vi "aggregator - viii - real - atomic.vi"(5 "aggregator action":T1, 7 "requested size":i32=20, 8 "number":dbl, 11 "state IN":T2={"Array "=[], "actual size"=0, "requested size"=20}) -> (0 "slope":dbl, 1 "interp average":dbl, 2 "mean":dbl, 3 "state OUT":T2={"Array "=[], "actual size"=0, "requested size"=20})   [LabVIEW 2021]
uses:
  interpolation state - real.ctl
  agregator -- action.ctl
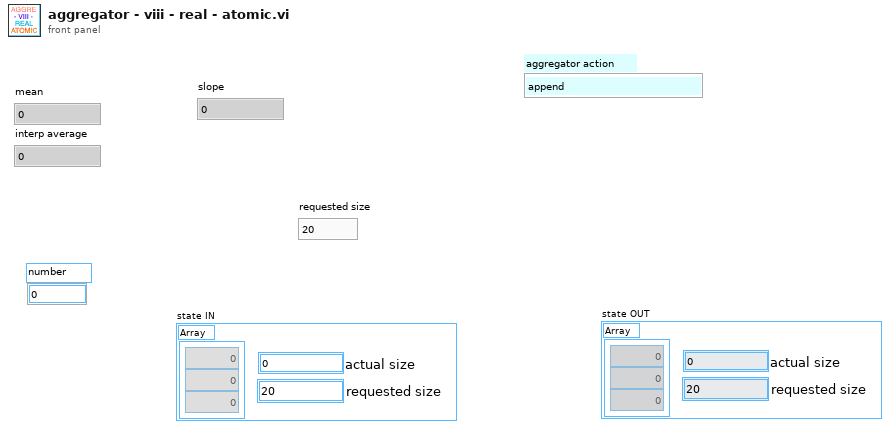
[diagram p1: front panel]
types:
  T1 = typedef "agregator -- action.ctl" = enum16{"append", "interpolate", "empty!", "force", "init", "scale", "read last"}
  T2 = typedef "interpolation state - real.ctl" = cluster{"Array ":dbl[], "actual size":i32, "requested size":i32}
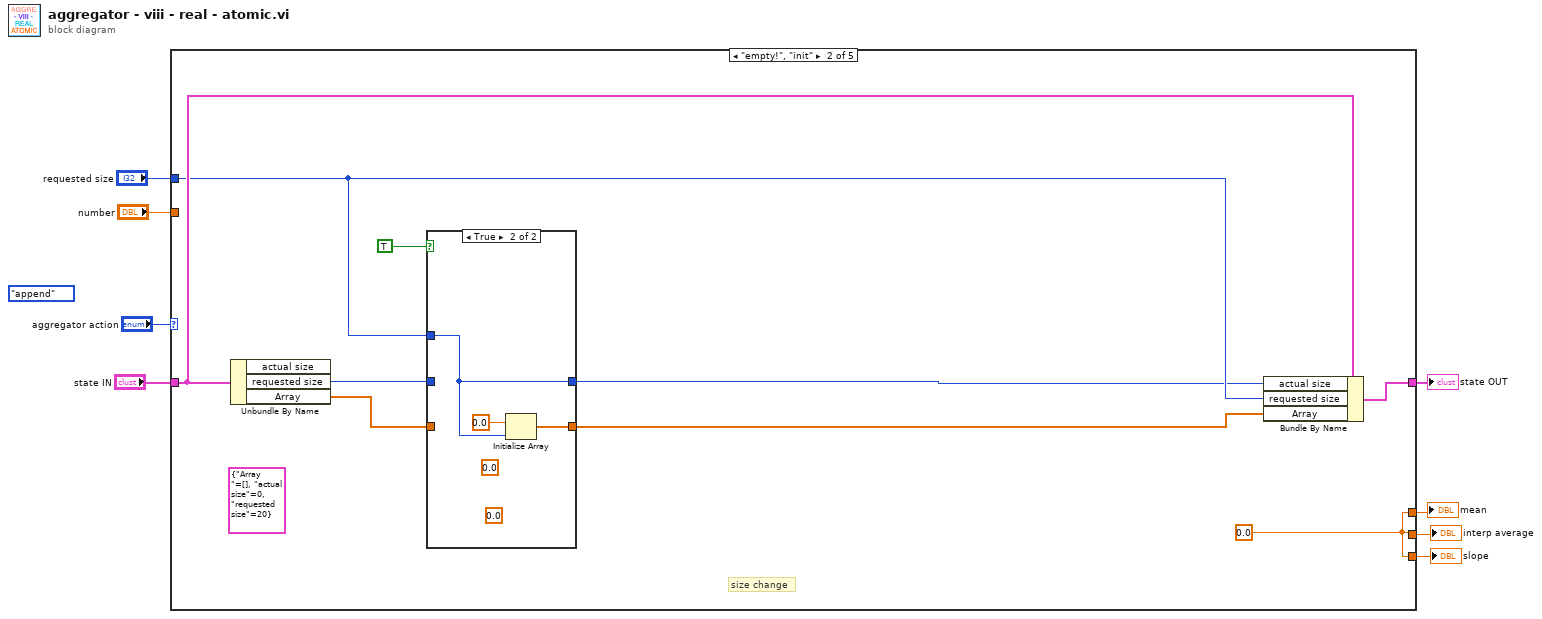
[diagram p0: block diagram]
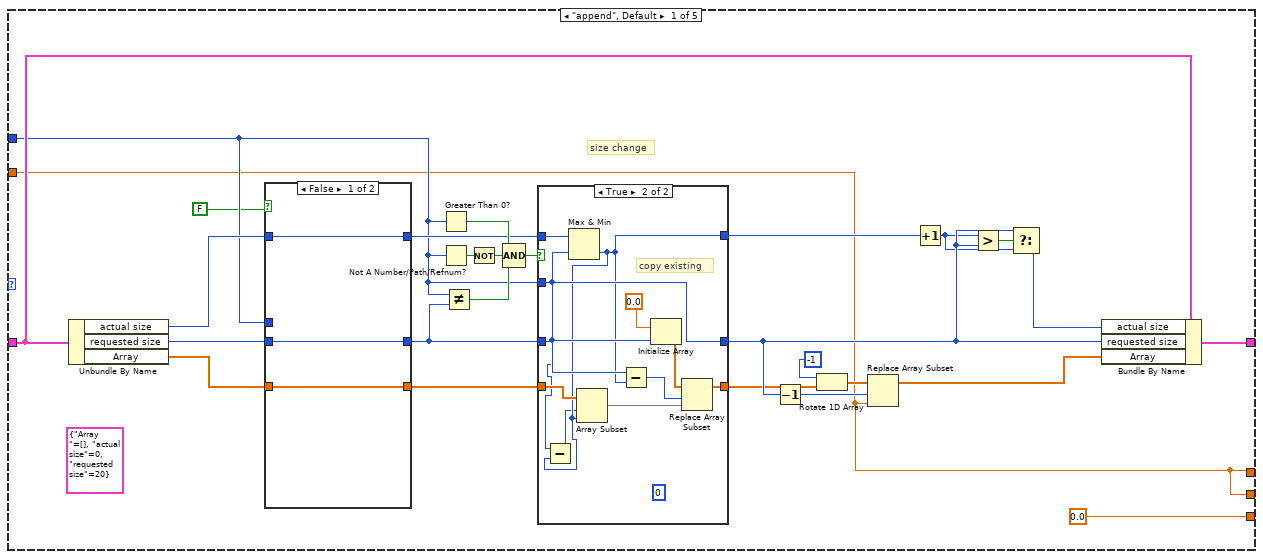
[diagram p2: hidden frame]
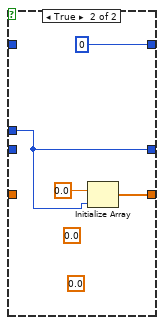
[diagram p4: hidden frame]
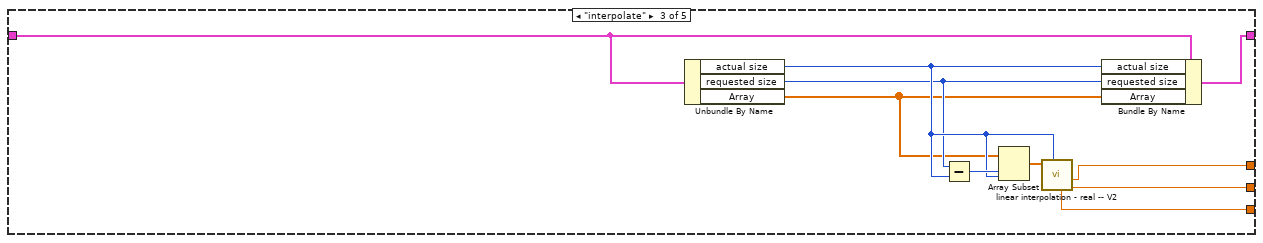
[diagram p6: hidden frame]
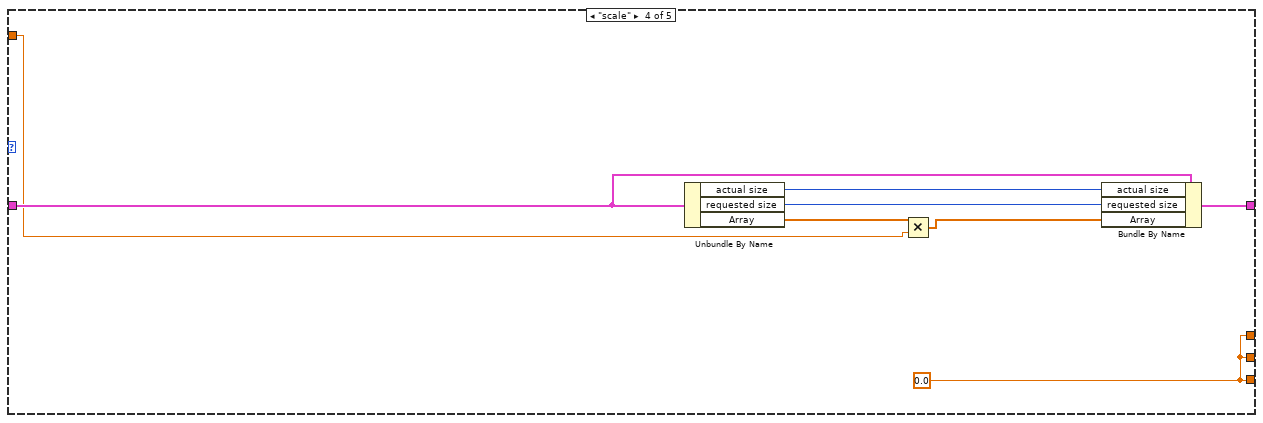
[diagram p7: hidden frame]
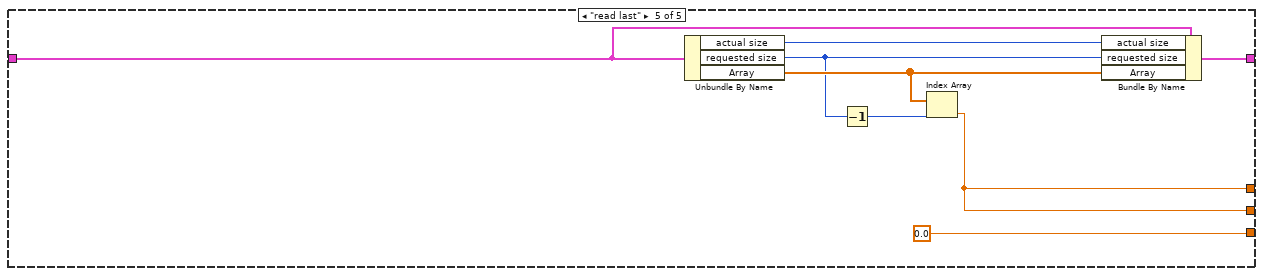
[diagram p8: hidden frame]
diagram:
  (unwired) agregator_--_action."append" ("aggregator action")
  n1 = case shown="\"empty!\", \"init\"" "aggregator action" {
    tunnel: [w9 w61 w80 w84 w89] -> w8
    tunnel: [w9 w61 w79 w84 w89] -> w7
    tunnel: [0.0 ("mean") w61 w78 w84 0.0 ("mean")] -> w6
    tunnel: [w32 w63 w77 w88 w96] -> w5
    tunnel: "state IN" -> [w31 w62 w76 w87 w95]
    tunnel: "number" -> [w9 _ _ w82 _]
    tunnel: "requested size" -> [w11 w58 _ _ _]
    frame "append", Default {
      (unwired) T2 {"Array "=[], "actual size"=0, "requested size"=20} ("Cluster")
      # "size change"
      n2 = Unbundle By Name(w31) -> ("actual size"=w34:i32, "requested size"=w35:i32, "Array"=w33:dbl[])
      n3 = case shown="False" FALSE {
        tunnel: w34 -> [w52 _]
        tunnel: [w52 0] -> w17
        tunnel: w33 -> [w50 _]
        tunnel: w11 -> [_ w53]
        tunnel: w35 -> [w51 _]
        tunnel: [w50 w54] -> w20
        tunnel: [w51 w53] -> w18
        frame False {
        }
        frame True {
          (unwired) 0.0
          (unwired) 0.0
          n4 = Initialize Array(0.0, w53) -> (w54:dbl[])
        }
      }
      n5 = Greater Than 0?(x=w11) -> (x > 0?=w24:bool)
      n6 = Not A Number/Path/Refnum?(number/path/refnum=w11) -> (NaN/Path/Refnum?=w25:bool)
      n7 = Not Equal?(x=w11, y=w18) -> (x != y?=w22:bool)
      n8 = Not(x=w25) -> (.not. x?=w23:bool)
      n9 = Compound Arithmetic op=AND(w24, w23, w22) -> (w21:bool)
      n10 = case shown="True" w21 {
        tunnel: [w38 w40] -> w16
        tunnel: w17 -> [w38 w48]
        tunnel: [w37 w44] -> w29
        tunnel: w18 -> [w37 w41]
        tunnel: [w36 w47] -> w19
        tunnel: w20 -> [w36 w43]
        tunnel: w11 -> [_ w44]
        frame False {
        }
        frame True {
          (unwired) 0 ("disabled index (col)")
          # "copy existing"
          n11 = Max & Min(x=w48, y=w44) -> (min(x,y)=w40:i32)  [unwired: 1 out]
          n12 = Subtract(x=w41, y=w40) -> (x-y=w39:i32)
          n13 = Array Subset(array=w43, index=w39, length=w40) -> (w42:dbl[])
          n14 = Subtract(x=w44, y=w40) -> (x-y=w45:i32)
          n15 = Initialize Array(0.0, w44) -> (w46:dbl[])
          n16 = Replace Array Subset(array=w46, new element=w42, index=w45) -> (w47:dbl[])
        }
      }
      n17 = Decrement(x=w29) -> (x-1=w14:i32)
      n18 = Rotate 1D Array(1:w19, 2:-1 ("n")) -> (0:w13:dbl[])
      n19 = Replace Array Subset(array=w13, new element=w9, index=w14) -> (w28:dbl[])
      n20 = Increment(x=w16) -> (x+1=w26:i32)
      n21 = Greater?(x=w26, y=w29) -> (0:w27:bool)
      n22 = Select(t=w29, s=w27, f=w26) -> (s? t:f=w30:i32)
      n23 = Bundle By Name(cluster=w31, "actual size"=w30, "requested size"=w29, "Array"=w28) -> (w32:T2)
    }
    frame "empty!", "init" {
      w61 = 0.0 ("mean")
      (unwired) T2 {"Array "=[], "actual size"=0, "requested size"=20} ("Cluster")
      # "size change"
      n24 = Unbundle By Name(w62) -> ("requested size"=w65:i32, "Array"=w64:dbl[])  [unwired: 1 out]
      n25 = case shown="True" TRUE {
        tunnel: w64 -> [w66 _]
        tunnel: w58 -> [_ w68]
        tunnel: w65 -> [w67 _]
        tunnel: [w66 w69] -> w59
        tunnel: [w67 w68] -> w57
        frame False {
        }
        frame True {
          (unwired) 0.0
          (unwired) 0.0
          n26 = Initialize Array(0.0, w68) -> (w69:dbl[])
        }
      }
      n27 = Bundle By Name(cluster=w62, "actual size"=w57, "requested size"=w58, "Array"=w59) -> (w63:T2)
    }
    frame "interpolate" {
      n28 = Unbundle By Name(w76) -> ("actual size"=w73:i32, "requested size"=w72:i32, "Array"=w71:dbl[])
      n29 = Subtract(x=w72, y=w73) -> (x-y=w75:i32)
      n30 = Array Subset(array=w71, index=w75, length=w73) -> (w74:dbl[])
      n31 = call "linear interpolation - real -- V2.vi"("n"=w73, "Array"=w74) -> ("interpolated average"=w79:dbl, "mean"=w80:dbl, "slope"=w78:dbl)  [unwired: 4 in, 3 out]
      n32 = Bundle By Name(cluster=w76, "actual size"=w73, "requested size"=w72, "Array"=w71) -> (w77:T2)
    }
    frame "scale" {
      w84 = 0.0 ("mean")
      n33 = Unbundle By Name(w87) -> ("actual size"=w86:i32, "requested size"=w85:i32, "Array"=w83:dbl[])
      n34 = Multiply(x=w83, y=w82) -> (x*y=w81:dbl[])
      n35 = Bundle By Name(cluster=w87, "actual size"=w86, "requested size"=w85, "Array"=w81) -> (w88:T2)
    }
    frame "read last" {
      n36 = Unbundle By Name(w95) -> ("actual size"=w94:i32, "requested size"=w91:i32, "Array"=w92:dbl[])
      n37 = Decrement(x=w91) -> (x-1=w90:i32)
      n38 = Index Array(array=w92, index=w90) -> (element=w89:dbl)
      n39 = Bundle By Name(cluster=w95, "actual size"=w94, "requested size"=w91, "Array"=w92) -> (w96:T2)
    }
  }
  "mean" <- w8
  "interp average" <- w7
  "slope" <- w6
  "state OUT" <- w5
